vi "Stop.vi"(8 "error in (no error)":errorcluster, 11 "TrialBasedExperiment in":refnum<class "TrialBasedExperiment.lvclass">) -> (0 "error out":errorcluster, 3 "TrialBasedExperiment out":refnum<class "TrialBasedExperiment.lvclass">)   [LabVIEW 2011, in "TrialBasedExperiment.lvclass"]
uses:
  TrialBasedExperiment.lvclass
  Acquisition/Database/StimulationPrimary.ctl
  Acquisition/AcquistionObject/AcquistionObject.lvclass
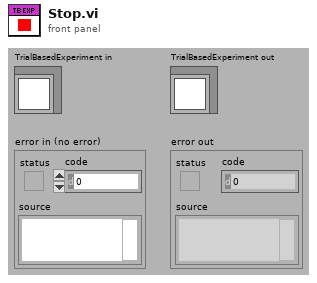
[diagram p1: front panel]
types:
  T1 = typedef "StimulationPrimary.ctl" = cluster{"setup":u8, "subject_id":i32, "session_start_time":dbl, "stim_start_time":dbl}
  T2 = cluster{"TotalTrials":u32, "Correct Trials":u32, "Incorrect Trials":u32, "Aborted Trials":u32}
  T3 = cluster{"TotalTrials":u32, "Correct Trials":u32, "Incorrect Trials":u32, "Scaled timestamp":dbl}
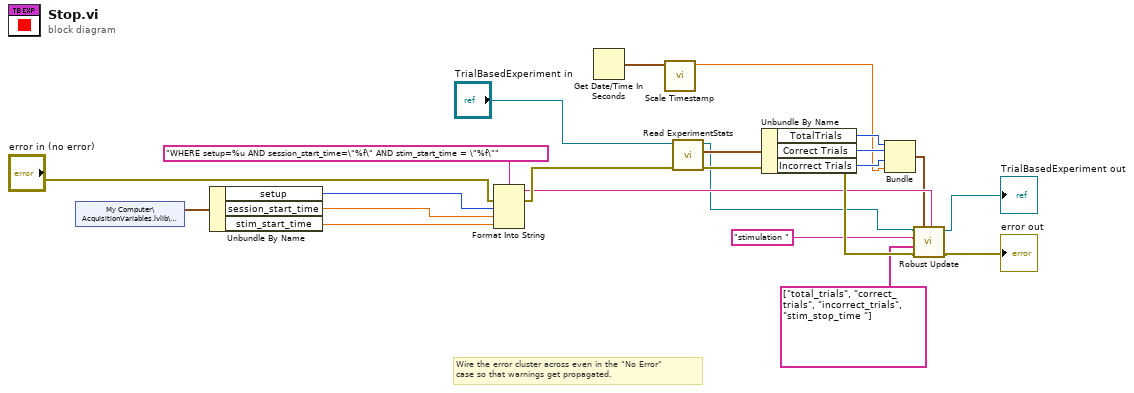
[diagram p0: block diagram]
diagram:
  # "Wire the error cluster across even in the \"No Error\"\ncase so that warnings get propagated."
  n1 = shared-variable "My Computer\\AcquisitionVariables.lvlib\\StimulationPK"() -> (w22:T1)  [unwired: 1 in, 1 out]
  n2 = Unbundle By Name(w22) -> ("setup"=w20:u8, "session_start_time"=w14:dbl, "stim_start_time"=w13:dbl)
  n3 = Format Into String(format string="WHERE setup=%u AND session_start_time=\"%f\" AND stim_start_time = \"%f\"", error in="error in (no error)", w20, w14, w13) -> (resulting string=w4:string, error out=w5:errorcluster)  [unwired: 1 in]
  n4 = Get Date/Time In Seconds() -> (seconds since 1Jan1904=w12:timestamp)
  n5 = call "Scale Timestamp.vi"("Time Stamp"=w12) -> ("Scaled timestamp"=w11:dbl)  [unwired: 10 in]
  n6 = call-dynamic "Read ExperimentStats.vi"("error in (no error)"=w5, "TrialBasedExperiment in"="TrialBasedExperiment in") -> ("error out"=w9:errorcluster, "ExperimentStats"=w18:T2, "TrialBasedExperiment out"=w2:refnum<class "TrialBasedExperiment.lvclass">)  [unwired: 7 in]
  n7 = Unbundle By Name(w18) -> ("TotalTrials"=w17:u32, "Correct Trials"=w16:u32, "Incorrect Trials"=w15:u32)
  n8 = Bundle("TotalTrials"=w17, "Correct Trials"=w16, "Incorrect Trials"=w15, "Scaled timestamp"=w11) -> (w3:T3)  [unwired: 1 in]
  n9 = call "Robust Update.vi"("condition"=w4, "data"=w3, "error in (no error)"=w9, "columns"=string[] ["total_trials", "correct_trials", "incorrect_trials", "stim_stop_time "], "table"="stimulation ", "AcquistionObject.lvclass"=w2) -> ("error out"=→"error out":errorcluster, "AcquistionObject out"=→"TrialBasedExperiment out":refnum<class "TrialBasedExperiment.lvclass">)  [unwired: 4 in]
